vi "Allocate Buffer.vi"(0 "camHandle IN":u32, 2 "Allocated Frames":u32=16, 11 "Error IN":errorcluster) -> (4 "buffHandle OUT":u32, 15 "Error OUT":errorcluster)   [LabVIEW 2020]
uses:
  Desktop/Vision Point LabVIEW/KYFGLib_lv.lvlib
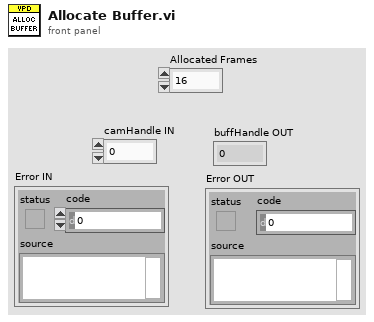
[diagram p1: front panel]
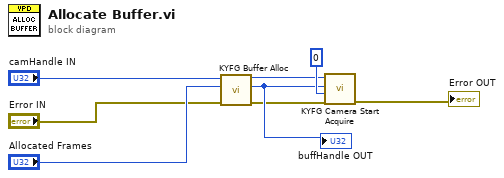
[diagram p0: block diagram]
diagram:
  n1 = call "KYFG Buffer Alloc.vi"("error in (no error)"="Error IN", "frames"="Allocated Frames", "camHandle"="camHandle IN") -> ("error out"=w4:errorcluster, "buffHandle"=w5:u32, "camHandle out"=w6:u32)  [unwired: 6 in]
  "buffHandle OUT" <- w5
  n2 = call "KYFG Camera Start Acquire.vi"("error in (no error)"=w4, "frames"=u32 0, "buffHandle"=w5, "camHandle"=w6) -> ("error out"=→"Error OUT":errorcluster)  [unwired: 5 in, 2 out]
